vi "robot1.vi"() -> ()   [LabVIEW 2010]
uses:
  <vilib>/Analysis/Matrix/Datatypes/RealMatrix.ctl
  <vilib>/robotics/Kinematics/Link/Joint Type.ctl
  <vilib>/robotics/Kinematics/Link/NI_Robotics_Link.lvclass
  <vilib>/robotics/Kinematics/Robot/NI_Robotics_Serial Robot Arm.lvclass
  <vilib>/robotics/Kinematics/Robot/Forward Kinematics (Point).vi
  <vilib>/robotics/Kinematics/Plotting/NI_Robotics_3DKinematics.lvlib
  <vilib>/robotics/Kinematics/NI_Kinematics.lvlib
  <vilib>/Analysis/Matrix/NI_Matrix.lvlib
panel:
  out "end effector transform":T1
  out "16bit integer 4":i16
  out "16bit integer 3":i16
  out "16bit integer 2":i16
  out "16bit integer":i16
  in  "Control":dbl[](array[slide]) scale=-90.0..90.0
  in  "stop":bool
  out "3D Picture Control":refnum<vi>(3d-picture)
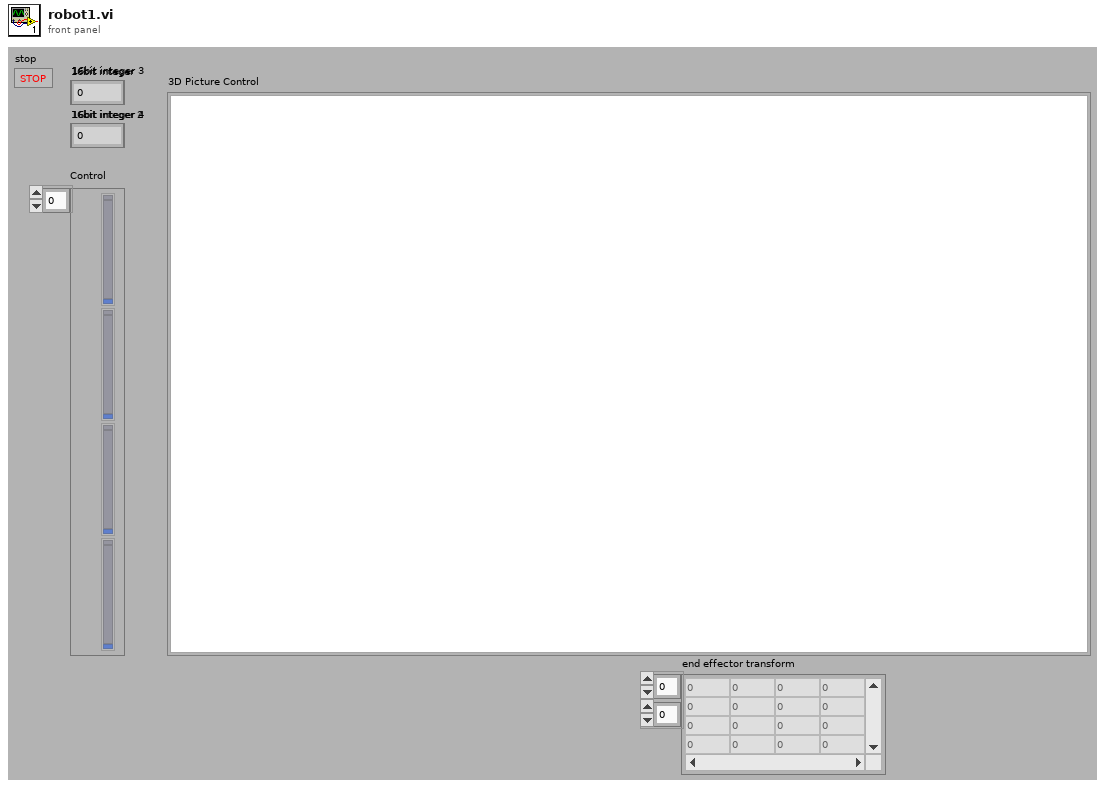
[diagram p1: front panel]
types:
  T1 = typedef "NI_Matrix.lvlib/RealMatrix.ctl" = dbl[][]
  T2 = typedef "NI_Robotics_Link.lvclass/Joint Type.ctl" = enum16{"Revolute", "Prismatic"}
  T3 = cluster{"twist angle":dbl, "length":dbl, "rotation angle":dbl, "offset distance":dbl, "joint type":T2, "joint coordinate offset":dbl}
  T4 = cluster{"Control[0]":dbl, "Control[1]":dbl, "Control[2]":dbl, "Control[3]":dbl, "Control[4]":dbl, "Control[5]":dbl, "Control[6]":dbl, "Control[7]":dbl, "Control[8]":dbl}
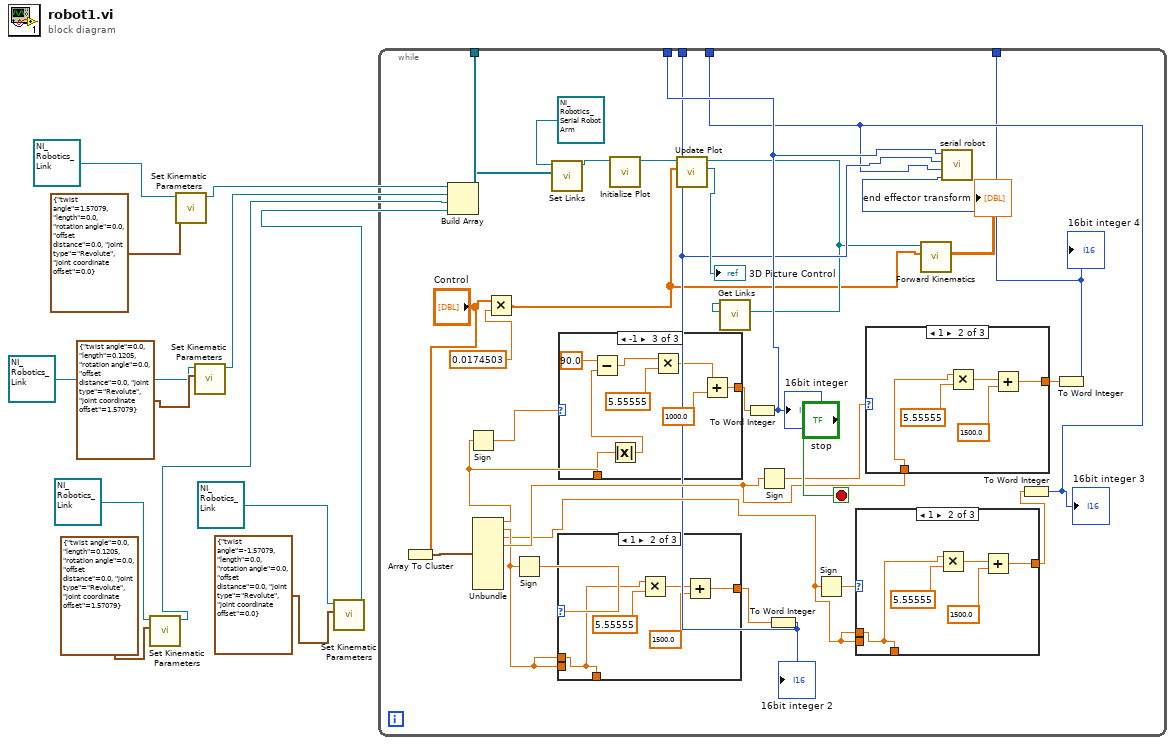
[diagram p0: block diagram]
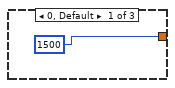
[diagram p2: hidden frame]
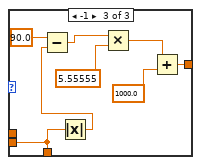
[diagram p3: hidden frame]
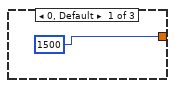
[diagram p4: hidden frame]
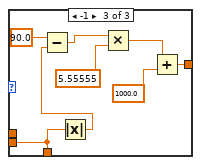
[diagram p5: hidden frame]
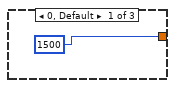
[diagram p6: hidden frame]
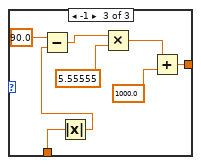
[diagram p7: hidden frame]
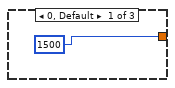
[diagram p8: hidden frame]
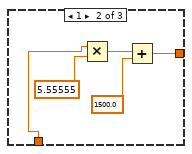
[diagram p9: hidden frame]
diagram:
  n1 = call <vilib>:"Set Kinematic Parameters.vi"("kinematic parameters"=T3 {"twist angle"=0.0, "length"=0.1205, "rotation angle"=0.0, "offset distance"=0.0, "joint type"=enum."Revolute", "joint coordinate offset"=1.57079}, "link in"=refnum<class "NI_Robotics_Link.lvclass"> refnum) -> ("link out"=w2:refnum<class "NI_Robotics_Link.lvclass">)  [unwired: 8 in, 1 out]
  n2 = call <vilib>:"Set Kinematic Parameters.vi"("kinematic parameters"=T3 {"twist angle"=1.57079, "length"=0.0, "rotation angle"=0.0, "offset distance"=0.0, "joint type"=enum."Revolute", "joint coordinate offset"=0.0}, "link in"=refnum<class "NI_Robotics_Link.lvclass"> refnum) -> ("link out"=w11:refnum<class "NI_Robotics_Link.lvclass">)  [unwired: 8 in, 1 out]
  n3 = call <vilib>:"Set Kinematic Parameters.vi"("kinematic parameters"=T3 {"twist angle"=0.0, "length"=0.1205, "rotation angle"=0.0, "offset distance"=0.0, "joint type"=enum."Revolute", "joint coordinate offset"=1.57079}, "link in"=refnum<class "NI_Robotics_Link.lvclass"> refnum) -> ("link out"=w7:refnum<class "NI_Robotics_Link.lvclass">)  [unwired: 8 in, 1 out]
  n4 = call <vilib>:"Set Kinematic Parameters.vi"("kinematic parameters"=T3 {"twist angle"=-1.57079, "length"=0.0, "rotation angle"=0.0, "offset distance"=0.0, "joint type"=enum."Revolute", "joint coordinate offset"=0.0}, "link in"=refnum<class "NI_Robotics_Link.lvclass"> refnum) -> ("link out"=w1:refnum<class "NI_Robotics_Link.lvclass">)  [unwired: 8 in, 1 out]
  n5 = Build Array(w11, w7, w2, w1) -> (w10:refnum<class "NI_Robotics_Link.lvclass">[])
  n6 = while {
    tunnel: w10 -> [w41]
    tunnel: [w20] -> _
    tunnel: [w19] -> _
    tunnel: [w18] -> _
    tunnel: [w17] -> _
    stop <- "stop" stop-if-true
    n7 = Array To Cluster(array="Control") -> (cluster=w33:T4)
    n8 = Unbundle(w33) -> ("Control[0]"=w31:dbl, "Control[1]"=w22:dbl, "Control[2]"=w21:dbl, "Control[3]"=w24:dbl)  [unwired: 5 out]
    n9 = Sign(1:w31) -> (0:w32:dbl)
    n10 = Multiply(x="Control", y=0.0174503) -> (x*y=w15:dbl[])
    n11 = Sign(1:w22) -> (0:w29:dbl)
    n12 = call <vilib>:"Set Links.vi"("links"=w41, "serial arm in"=refnum<class "NI_Robotics_Serial Robot Arm.lvclass"> refnum) -> ("serial arm out"=w39:refnum<class "NI_Robotics_Serial Robot Arm.lvclass">)  [unwired: 8 in, 1 out]
    n13 = case shown="1" w29 {
      tunnel: [_ w43 w48] -> _
      tunnel: [1500 w44 w49] -> w28
      tunnel: w22 -> [_ _ w48]
      tunnel: w22 -> [_ w43 _]
      frame 0, Default {
      }
      frame 1 {
        n14 = Multiply(x=w43, y=5.55555) -> (x*y=w46:dbl)
        n15 = Add(x=w46, y=1500.0) -> (x+y=w44:dbl)
      }
      frame -1 {
        n16 = Absolute Value(x=w48) -> (abs(x)=w53:dbl)
        n17 = Subtract(x=90.0, y=w53) -> (x-y=w50:dbl)
        n18 = Multiply(x=w50, y=5.55555) -> (x*y=w55:dbl)
        n19 = Add(x=w55, y=1000.0) -> (x+y=w49:dbl)
      }
    }
    n20 = case shown="-1" w32 {
      tunnel: w31 -> [_ w85 w95]
      tunnel: [1500 w86 w90] -> w30
      frame 0, Default {
      }
      frame 1 {
        n21 = Multiply(x=w85, y=5.55555) -> (x*y=w88:dbl)
        n22 = Add(x=w88, y=1500.0) -> (x+y=w86:dbl)
      }
      frame -1 {
        n23 = Absolute Value(x=w95) -> (abs(x)=w94:dbl)
        n24 = Subtract(x=90.0, y=w94) -> (x-y=w91:dbl)
        n25 = Multiply(x=w91, y=5.55555) -> (x*y=w97:dbl)
        n26 = Add(x=w97, y=1000.0) -> (x+y=w90:dbl)
      }
    }
    n27 = call <vilib>:"Initialize Plot.vi"("serial arm in"=w39) -> ("serial arm out"=w37:refnum<class "NI_Robotics_Serial Robot Arm.lvclass">)  [unwired: 9 in, 1 out]
    n28 = call <vilib>:"Update Plot.vi"("joint positions"=w15, "serial arm in"=w37) -> ("serial arm scene"=→"3D Picture Control":refnum<vi>, "serial arm out"=w16:refnum<class "NI_Robotics_Serial Robot Arm.lvclass">)  [unwired: 7 in, 1 out]
    n29 = call <vilib>:"Get Links.vi"("serial arm in"=w16) -> ()  [unwired: 8 in, 3 out]
    n30 = To Word Integer(number=w30) -> (16bit integer=w20:i16)
    "16bit integer" <- w20
    n31 = Sign(1:w24) -> (0:w25:dbl)
    n32 = To Word Integer(number=w28) -> (16bit integer=w19:i16)
    "16bit integer 2" <- w19
    n33 = Sign(1:w21) -> (0:w27:dbl)
    n34 = case shown="1" w27 {
      tunnel: [_ w57 w62] -> _
      tunnel: [1500 w58 w63] -> w26
      tunnel: w21 -> [_ _ w62]
      tunnel: w21 -> [_ w57 _]
      frame 0, Default {
      }
      frame 1 {
        n35 = Multiply(x=w57, y=5.55555) -> (x*y=w60:dbl)
        n36 = Add(x=w60, y=1500.0) -> (x+y=w58:dbl)
      }
      frame -1 {
        n37 = Absolute Value(x=w62) -> (abs(x)=w67:dbl)
        n38 = Subtract(x=90.0, y=w67) -> (x-y=w64:dbl)
        n39 = Multiply(x=w64, y=5.55555) -> (x*y=w69:dbl)
        n40 = Add(x=w69, y=1000.0) -> (x+y=w63:dbl)
      }
    }
    n41 = case shown="1" w25 {
      tunnel: w24 -> [_ w71 w81]
      tunnel: [1500 w72 w76] -> w23
      frame 0, Default {
      }
      frame 1 {
        n42 = Multiply(x=w71, y=5.55555) -> (x*y=w74:dbl)
        n43 = Add(x=w74, y=1500.0) -> (x+y=w72:dbl)
      }
      frame -1 {
        n44 = Absolute Value(x=w81) -> (abs(x)=w80:dbl)
        n45 = Subtract(x=90.0, y=w80) -> (x-y=w77:dbl)
        n46 = Multiply(x=w77, y=5.55555) -> (x*y=w83:dbl)
        n47 = Add(x=w83, y=1000.0) -> (x+y=w76:dbl)
      }
    }
    n48 = call-poly <vilib>:"Forward Kinematics.vi"("joint positions"=w15, "serial arm in"=w16) -> ("end effector transform"=→"end effector transform":T1)  [unwired: 7 in, 2 out]
    n49 = To Word Integer(number=w26) -> (16bit integer=w18:i16)
    "16bit integer 3" <- w18
    n50 = To Word Integer(number=w23) -> (16bit integer=w17:i16)
    "16bit integer 4" <- w17
    n51 = call "serial robot.vi"("Numeric"=w20, "Numeric 2"=w19, "Numeric 3"=w18, "Numeric 4"=w17) -> ()  [unwired: 7 in]
  }
